vi "Sample To use.vi"() -> ()   [LabVIEW 2014]
uses:
  Event_class/EventMsg.lvclass
panel:
  in  "Name":string
  out "Msg 3":string
  in  "stop":bool
  in  "Msg 2":string="q2333"
  out "Msg":string
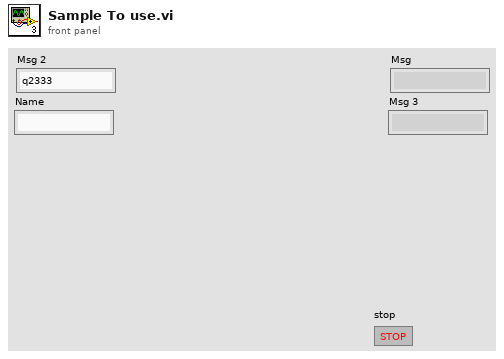
[diagram p1: front panel]
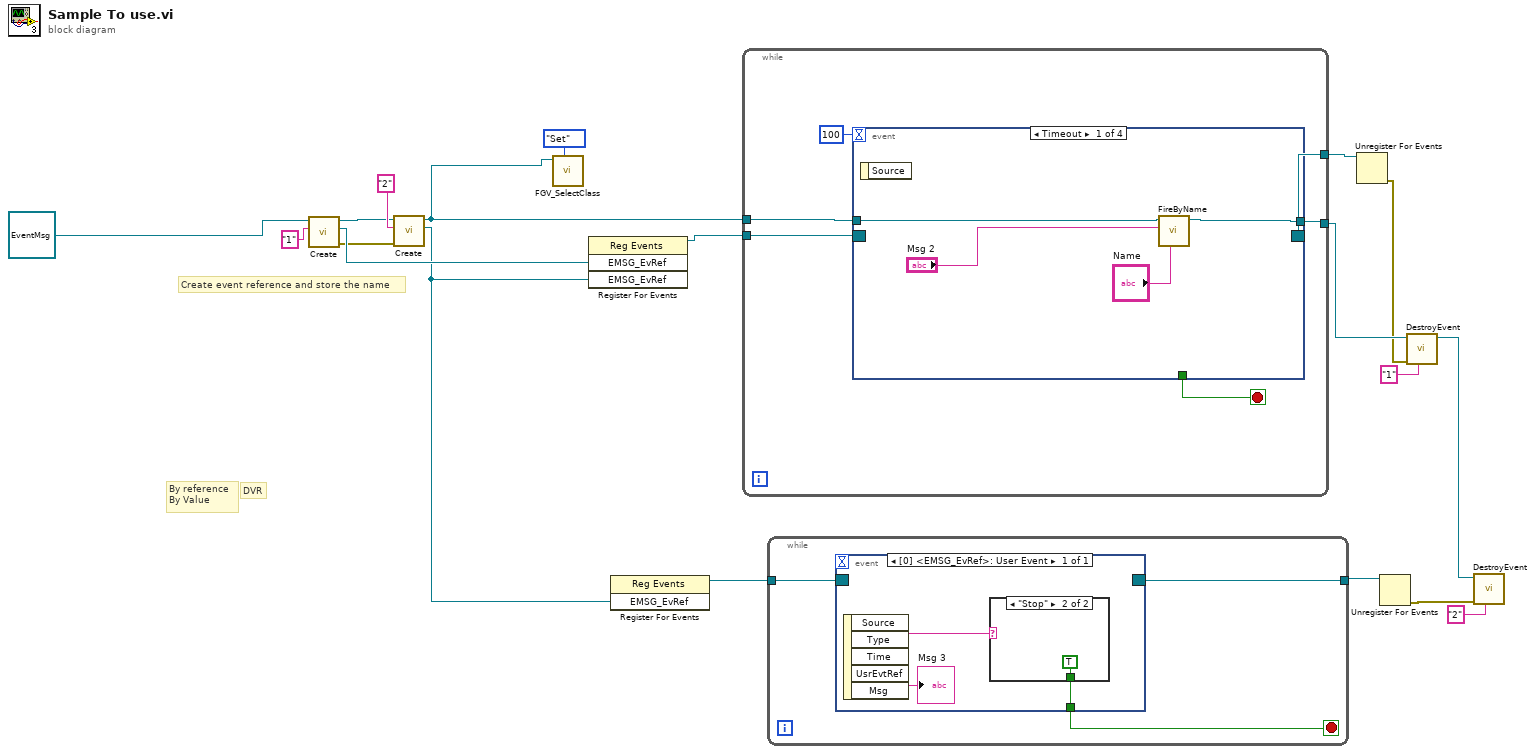
[diagram p0: block diagram]
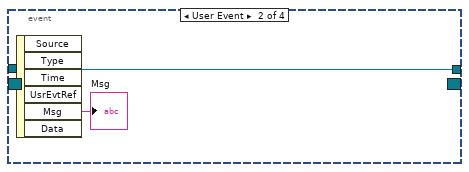
[diagram p3: hidden frame]
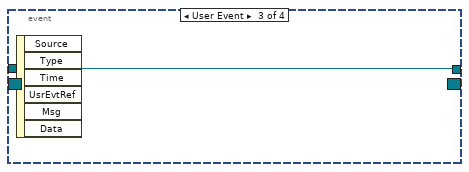
[diagram p4: hidden frame]
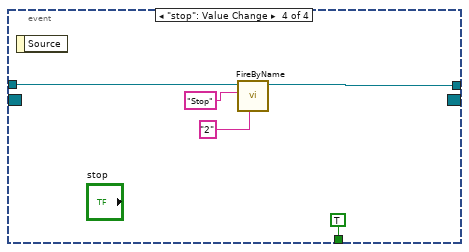
[diagram p5: hidden frame]
diagram:
  # "DVR"
  # "By reference \nBy Value"
  # "Create event reference and store the name"
  n1 = call-dynamic "Create.vi"("Name"="1", "object in"=refnum<class "EventMsg.lvclass"> refnum) -> ("error out"=w7:errorcluster, "EMSG_EvRef"=w16:refnum<user-event>, "object out"=w9:refnum<class "EventMsg.lvclass">)  [unwired: 7 in]
  n2 = call-dynamic "Create.vi"("error in (no error)"=w7, "Name"="2", "object in"=w9) -> ("EMSG_EvRef"=w4:refnum<user-event>, "object out"=w1:refnum<class "EventMsg.lvclass">)  [unwired: 6 in, 1 out]
  n3 = call "FGV_SelectClass.vi"("Action"=enum16{"Set", "Get"}."Set", "EventMsg.lvclass"=w1) -> ()  [unwired: 9 in, 1 out]
  n4 = register-events(w16, w4) -> (reference out=w17:refnum<event-registration>)  [unwired: 2 in, 1 out]
  n5 = register-events(w4) -> (reference out=w15:refnum<event-registration>)  [unwired: 2 in, 1 out]
  n6 = while {
    tunnel: w17 -> [w24]
    tunnel: w1 -> [w22]
    tunnel: [w21] -> w13
    tunnel: [w20] -> w12
    stop <- w25 stop-if-true
    n7 = event shown="[0] Timeout" {
      selector: w24 -> [_ _ _ _]
      dyn-events: [_ _ _ _] -> w20
      timeout: 100 -> [_ _ _ _]
      tunnel: w22 -> [w28 w30 w32 w35]
      tunnel: [_ _ _ TRUE ("stop")] -> w25
      tunnel: [w27 w30 w32 w34] -> w21
      event Timeout {
        n8 = event-data() -> ()  [unwired: 1 in, 1 out]
        n9 = call-dynamic "FireByName.vi"("Name"="Name", "Msg"="Msg 2", "object in"=w28) -> ("object out"=w27:refnum<class "EventMsg.lvclass">)  [unwired: 7 in, 1 out]
      }
      event User Event {
        n10 = event-data() -> ("Msg"=→"Msg":string)  [unwired: 1 in, 5 out]
      }
      event User Event {
        n11 = event-data() -> ()  [unwired: 1 in, 6 out]
      }
      event "stop": Value Change {
        n12 = event-data() -> ()  [unwired: 1 in, 1 out]
        n13 = call-dynamic "FireByName.vi"("Name"="2", "Msg"="Stop", "object in"=w35) -> ("object out"=w34:refnum<class "EventMsg.lvclass">)  [unwired: 7 in, 1 out]
      }
    }
  }
  n14 = while {
    tunnel: w15 -> [w40]
    tunnel: [w38] -> w14
    stop <- w39 stop-if-true
    n15 = event shown="[0] <EMSG_EvRef>: User Event" {
      selector: w40 -> [_]
      dyn-events: [_] -> w38
      timeout: _ -> [_]
      tunnel: [w41] -> w39
      event User Event {
        n16 = event-data() -> ("Msg"=w42:string)  [unwired: 1 in, 4 out]
        "Msg 3" <- w42
        n17 = case shown="\"Stop\"" w42 {
          tunnel: [_ TRUE] -> w41
          frame "False", Default {
          }
          frame "Stop" {
          }
        }
      }
    }
  }
  n18 = Unregister For Events(event registration refnum=w12) -> (error out=w11:errorcluster)  [unwired: 1 in]
  n19 = Unregister For Events(event registration refnum=w14) -> (error out=w10:errorcluster)  [unwired: 1 in]
  n20 = call-dynamic "DestroyEvent.vi"("Name"="1", "error in (no error)"=w11, "object in"=w13) -> ("object out"=w8:refnum<class "EventMsg.lvclass">)  [unwired: 7 in, 1 out]
  n21 = call-dynamic "DestroyEvent.vi"("Name"="2", "error in (no error)"=w10, "object in"=w8) -> ()  [unwired: 7 in, 2 out]
